vi "get information display strings.vi"(8 "error in":errorcluster, 11 "Abstract Instrument in":refnum<class "Abstract Instrument.lvclass">) -> (0 "error out":errorcluster, 1 "Data":string[](array[string]), 2 "Labels":string[](array[string]), 3 "Abstract Instrument out":refnum<class "Abstract Instrument.lvclass">)   [LabVIEW 2025, in "Abstract Engine.lvlib" / "Abstract Instrument.lvclass"]
doc: "Copyright 2017 National Instruments Corporation\n\nLicensed under the Apache License, Version 2.0 (the \"License\"); you may not use this file except in compliance with the License. You may obtain a copy of the License at http://www.apache.org/licenses/LICENSE-2.0\nUnless required by applicable law or agreed to in writing, software distributed under the License is distributed on an \"AS IS\" BASIS, WITHOUT WARRANTIES OR CONDITIONS OF ANY KIND, either express or implied. See the License for the specific language governing permissions and limitations under the License."
uses:
  Abstract Instrument.lvclass
  Abstract Instrument.lvclass/Abstract Instrument.ctl
  Read error cluster.vi
  Users/Public/Documents/Sandia National Labs/TSS Plugin/CEF.lvlibp/serializable configuration/CEF_serializable configuration.lvclass
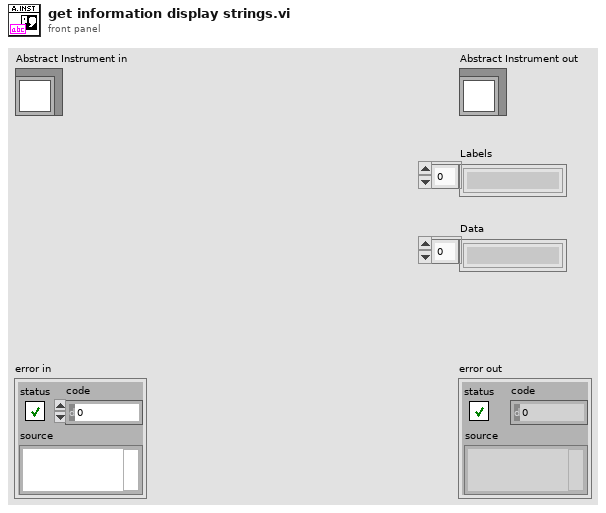
[diagram p1: front panel]
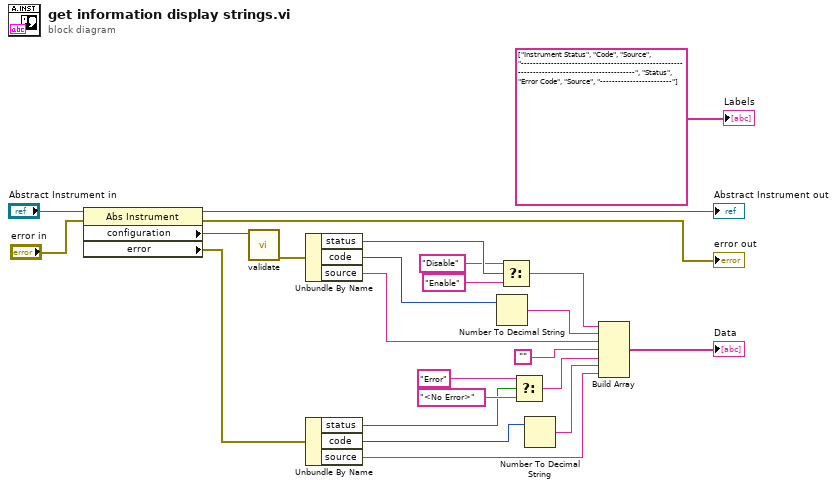
[diagram p0: block diagram]
diagram:
  n1 = property class="Abs Instrument"(reference="Abstract Instrument in", error in="error in") -> (reference out=→"Abstract Instrument out":refnum<class "Abstract Instrument.lvclass">, error out=→"error out":errorcluster, "configuration"=w22:refnum<class "CEF_serializable configuration.lvclass">, "error"=w20:errorcluster)
  n2 = call-dynamic "validate.vi"("CEF_Configuration in"=w22) -> ("error out"=w21:errorcluster)  [unwired: 9 in, 1 out]
  n3 = Unbundle By Name(w21) -> ("status"=w13:bool, "code"=w17:i32, "source"=w15:string)
  n4 = Unbundle By Name(w20) -> ("status"=w7:bool, "code"=w6:i32, "source"=w4:string)
  n5 = Number To Decimal String(number=w17) -> (decimal integer string=w16:string)  [unwired: 1 in]
  n6 = Select(t="Disable" ("String"), s=w13, f="Enable" ("String")) -> (s? t:f=w10:string)
  n7 = Select(t="Error" ("String"), s=w7, f="<No Error>" ("String")) -> (s? t:f=w2:string)
  n8 = Number To Decimal String(number=w6) -> (decimal integer string=w5:string)  [unwired: 1 in]
  n9 = Build Array(w10, w16, w15, "", w2, w5, w4) -> (→"Data":string[])
  "Labels" <- string[] ["Instrument Status", "Code", "Source", "---------------------------------------------------------------------------------------------", "Status", "Error Code", "Source", "------------------------"] ("Labels")
